vi "id.vi"(8 "error in (no error)":errorcluster, 11 "TestSuite in":refnum<class "TestSuite.lvclass">) -> (0 "error out":errorcluster, 1 "GUID":string, 2 "Description":string, 3 "TestSuite out":refnum<class "TestSuite.lvclass">)   [LabVIEW 2013, in "TestSuite.lvclass"]
uses:
  TestSuite.lvclass
  TestSuite.lvclass/TestSuite.ctl
  Libraries/VITesterUtilities.lvlib
panel:
  # "JKI VI Tester for LabVIEW\nhttp://jkisoft.com/vi-tester\nCopyright (C) 2007-2009, JKI <info@jkisoft.com>\nALL RIGHTS RESERVED"
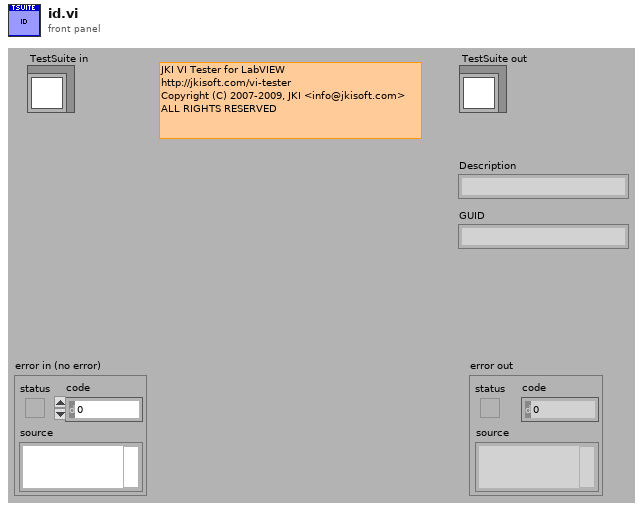
[diagram p1: front panel]
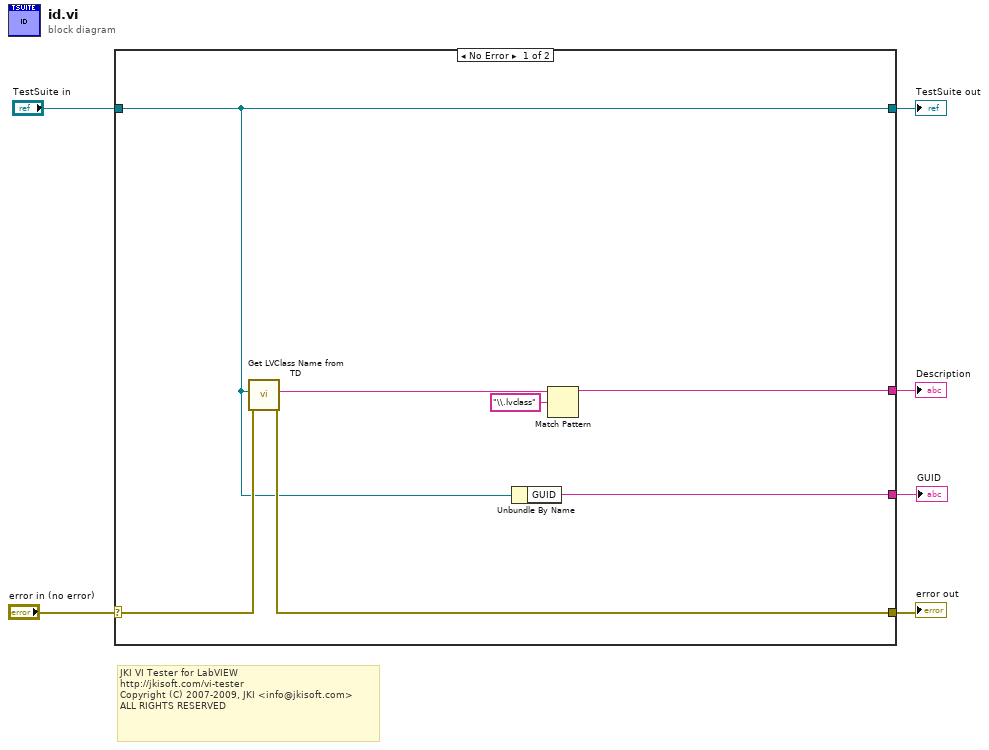
[diagram p0: block diagram]
diagram:
  # "JKI VI Tester for LabVIEW\nhttp://jkisoft.com/vi-tester\nCopyright (C) 2007-2009, JKI <info@jkisoft.com>\nALL RIGHTS RESERVED"
  n1 = case shown="No Error" "error in (no error)" {
    selector: "error in (no error)" -> [w13 w15]
    tunnel: [w9 w15] -> w5
    tunnel: [w8 w14] -> w3
    tunnel: "TestSuite in" -> [w8 w14]
    tunnel: [w10 _] -> w2
    tunnel: [w7 _] -> w1
    frame No Error {
      n2 = call "Get LVClass Name from TD.vi"("error in"=w13, "Variant"=w8) -> ("error out"=w9:errorcluster, "LVClass Name"=w11:string)  [unwired: 8 in]
      n3 = Unbundle By Name(w8) -> ("GUID"=w7:string)
      n4 = Match Pattern(string=w11, regular expression="\\.lvclass") -> (before substring=w10:string)  [unwired: 1 in, 3 out]
    }
    frame Error {
    }
  }
  "error out" <- w5
  "TestSuite out" <- w3
  "Description" <- w2
  "GUID" <- w1
